vi "medidor1.vi"() -> ()   [LabVIEW 2009]
panel:
  out "Numeric":dbl
  in  "Directorio scripts":path
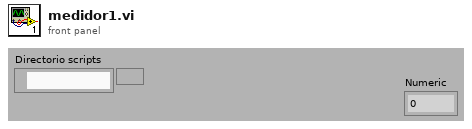
[diagram p1: front panel]
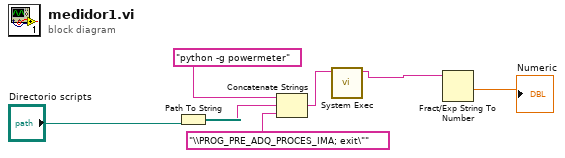
[diagram p0: block diagram]
diagram:
  n1 = Path To String(path="Directorio scripts") -> (string=w4:string)
  n2 = Concatenate Strings("python -g powermeter" ("command line"), w4, "\\PROG_PRE_ADQ_PROCES_IMA; exit\"" ("command line")) -> (w3:string)
  n3 = call <vilib>:"System Exec.vi"("command line"=w3) -> ("standard output"=w6:string)  [unwired: 7 in, 3 out]
  n4 = Fract/Exp String To Number(string=w6) -> (number=→"Numeric":dbl)  [unwired: 3 in, 1 out]
